vi "N5700 Initialize.vi"(0 "VISA name":refnum<visa-resource-name>="GPIB::5::INSTR", 2 "Timeout (3 sec)":u32=3, 5 "ID Query (T)":bool=TRUE, 7 "Reset (T)":bool=TRUE, 11 "error in (no error)":errorcluster) -> (4 "VISA out":refnum<visa-resource-name>, 15 "error out":errorcluster)   [LabVIEW 2020]
doc: "This VI passes the addressing information in \"VISA name\" and returns the instrument ID. You must run this VI before using any of the instrument driver VIs for this instrument.\n\nYou can optionally reset the instrument by setting the front panel reset control. \nYou can optionally read the instrument identity string and verify ithe instrument can be used with this driver.\n\nThe Timeout is seconds allowed for instrument to respond to data read. Default is 3 seconds.\n\nNotes:\n(1) This instrument driver supports IEEE-488, LAN and maybe USB ports. The \"VISA name\" input determines which port type and which instrument is initialized."
panel:
  # "Agilent Technologies  \nSeries N5700A\n  DC Power Supplies"
  # "Initialize Instrument\nOpen VISA Port"
  # "Seconds"
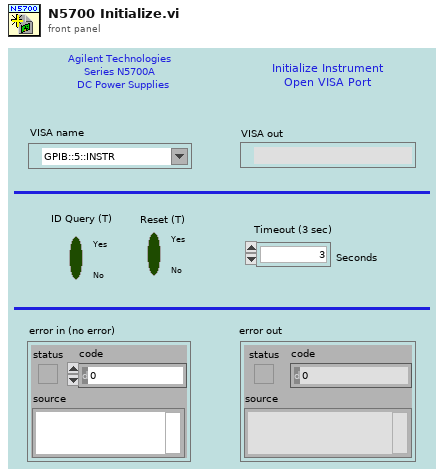
[diagram p1: front panel]
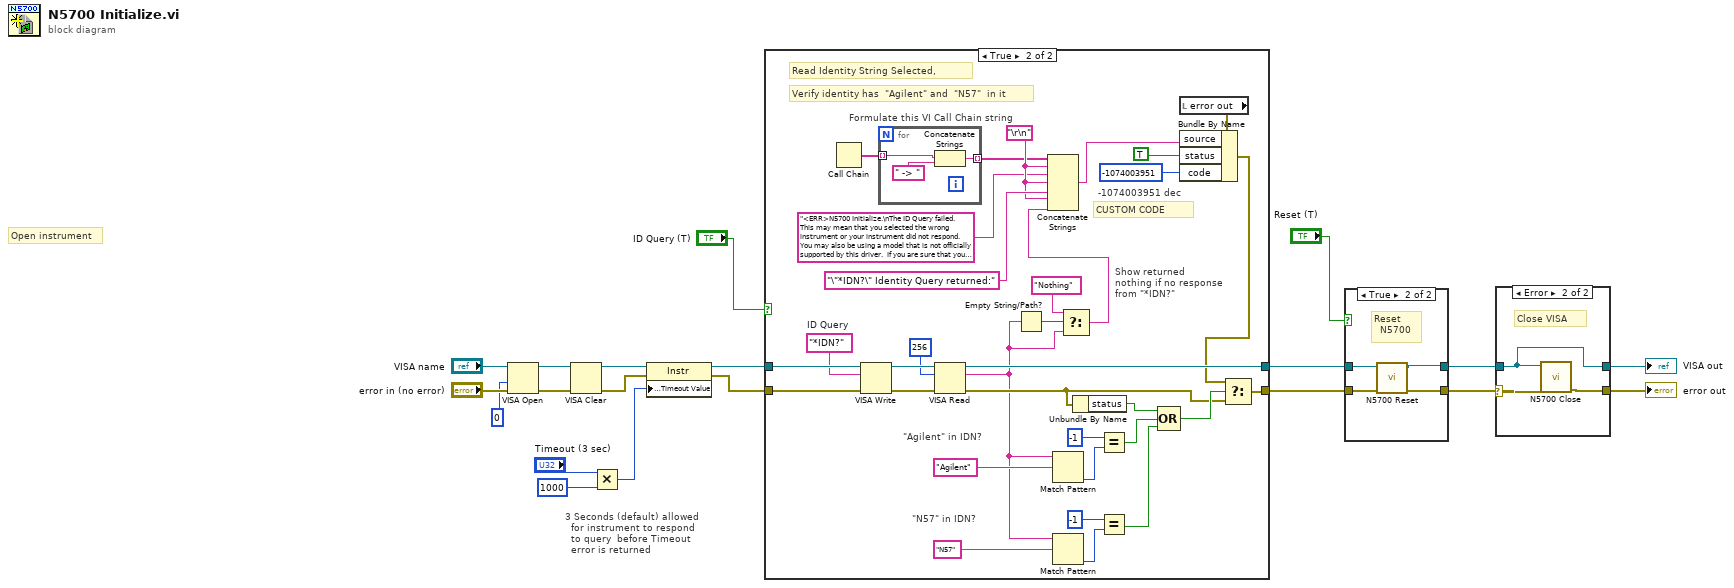
[diagram p0: block diagram]
diagram:
  # "3 Seconds (default) allowed\n  for instrument to respond \n  to query  before Timeout\n  error is returned"
  # "Open instrument"
  n1 = VISA Open(access mode=u32 0, error in (no error)="error in (no error)", VISA resource name="VISA name") -> (VISA resource name=w10:refnum<visa-resource-name>, error out=w9:errorcluster)  [unwired: 2 in]
  n2 = VISA Clear(VISA resource name=w10, error in (no error)=w9) -> (VISA resource name out=w8:refnum<visa-resource-name>, error out=w7:errorcluster)
  n3 = Multiply(x="Timeout (3 sec)", y=u32 1000) -> (x*y=w1:u32)
  n4 = property class="Instr"(reference=w8, error in=w7, "General Settings:Timeout Value"=w1) -> (reference out=w6:refnum<visa-resource-name>, error out=w5:errorcluster)
  n5 = case shown="True" "ID Query (T)" {
    tunnel: [w21 w55] -> w19
    tunnel: [w22 w52] -> w20
    tunnel: w6 -> [w22 w53]
    tunnel: w5 -> [w21 w54]
    frame False {
      # "Do Not Read Identity String"
    }
    frame True {
      w31 = "\r\n"
      w45 = "*IDN?"  # ID Query
      # "Show returned\nnothing if no response\nfrom \"*IDN?\""
      # "Formulate this VI Call Chain string"
      # "-1074003951 dec"
      # "CUSTOM CODE"
      # "\"N57\" in IDN?"
      # "\"Agilent\" in IDN?"
      # "Verify identity has  \"Agilent\" and  \"N57\"  in it"
      # "Read Identity String Selected,"
      n6 = Call Chain() -> (call chain=w30:string[])
      n7 = VISA Write(VISA resource name=w53, write buffer=w45, error in (no error)=w54) -> (VISA resource name out=w51:refnum<visa-resource-name>, error out=w50:errorcluster)  [unwired: 1 out]
      n8 = for {
        tunnel: w30 -> [w58] mode=indexing
        tunnel: [w56] -> w29 mode=indexing
        n9 = Concatenate Strings(w58, " -> ") -> (w56:string)
      }
      n10 = VISA Read(VISA resource name=w51, byte count=u32 256, error in (no error)=w50) -> (VISA resource name out=w52:refnum<visa-resource-name>, read buffer=w25:string, error out=w37:errorcluster)  [unwired: 1 out]
      n11 = Empty String/Path?(string/path=w25) -> (empty?=w26:bool)
      n12 = Match Pattern(string=w25, regular expression="Agilent") -> (offset past match=w47:i32)  [unwired: 1 in, 3 out]
      n13 = Match Pattern(string=w25, regular expression="N57") -> (offset past match=w44:i32)  [unwired: 1 in, 3 out]
      n14 = Select(t="Nothing" ("Source"), s=w26, f=w25) -> (s? t:f=w23:string)
      n15 = Concatenate Strings(w29, w31, "<ERR>N5700 Initialize.\nThe ID Query failed.  This may mean that you selected the wrong instrument or your instrument did not respond.  You may also be using a model that is not officially supported by this driver.  If you are sure that you have selected the correct instrument and it is responding, try disabling the ID Query." ("Source (VI Name)"), w31, "\"*IDN?\" Identity Query returned:" ("Source"), w31, w23) -> (w32:string)
      n16 = Unbundle By Name(w37) -> ("status"=w41:bool)
      n17 = Equal?(x=-1, y=w47) -> (x = y?=w40:bool)
      n18 = Equal?(x=-1, y=w44) -> (x = y?=w39:bool)
      n19 = Compound Arithmetic op=OR(w41, w40, w39) -> (w38:bool)
      n20 = local read "error out"() -> (w33:errorcluster)
      n21 = Bundle By Name(cluster=w33, "source"=w32, "status"=TRUE, "code"=-1074003951) -> (w28:errorcluster)
      n22 = Select(t=w28, s=w38, f=w37) -> (s? t:f=w55:errorcluster)
    }
  }
  n23 = case shown="True" "Reset (T)" {
    tunnel: w19 -> [w59 w63]
    tunnel: [w59 w61] -> w4
    tunnel: w20 -> [w60 w64]
    tunnel: [w60 w62] -> w16
    frame False {
      # "Do Not\n  Reset"
    }
    frame True {
      # "Reset  \n  N5700"
      n24 = call "N5700 Reset.vi"("error"=w63, "VISA"=w64) -> ("error out"=w61:errorcluster, "VISA out"=w62:refnum<visa-resource-name>)  [unwired: 5 in]
    }
  }
  n25 = case shown="Error" w4 {
    selector: w4 -> [w65 w69]
    tunnel: w16 -> [w66 w67]
    tunnel: [w66 w67] -> w15
    tunnel: [w65 w68] -> w14
    frame No Error {
    }
    frame Error {
      # "Close VISA"
      n26 = call "N5700 Close.vi"("error"=w69, "VISA name"=w67) -> ("error out"=w68:errorcluster)  [unwired: 6 in]
    }
  }
  "VISA out" <- w15
  "error out" <- w14
